vi "Abort.vi"   [LabVIEW 2023]
uses:
  <vilib>/eio/EIONode/EIONode.xnode
  <vilib>/rvi/DataTransferAndStorage/Container/XNode/niFpgaContainer.xnode
  <vilib>/rvi/DataTransferAndStorage/Register/Emulation/niFpgaRegisterEmulation.vi
  <vilib>/rvi/eio/common/nirviEmuTemplateMethod_errors.vi
types:
  T1 = cluster{bool, bool, bool, bool, bool, bool, bool, bool, bool, bool, bool, bool, bool, bool, bool, bool}
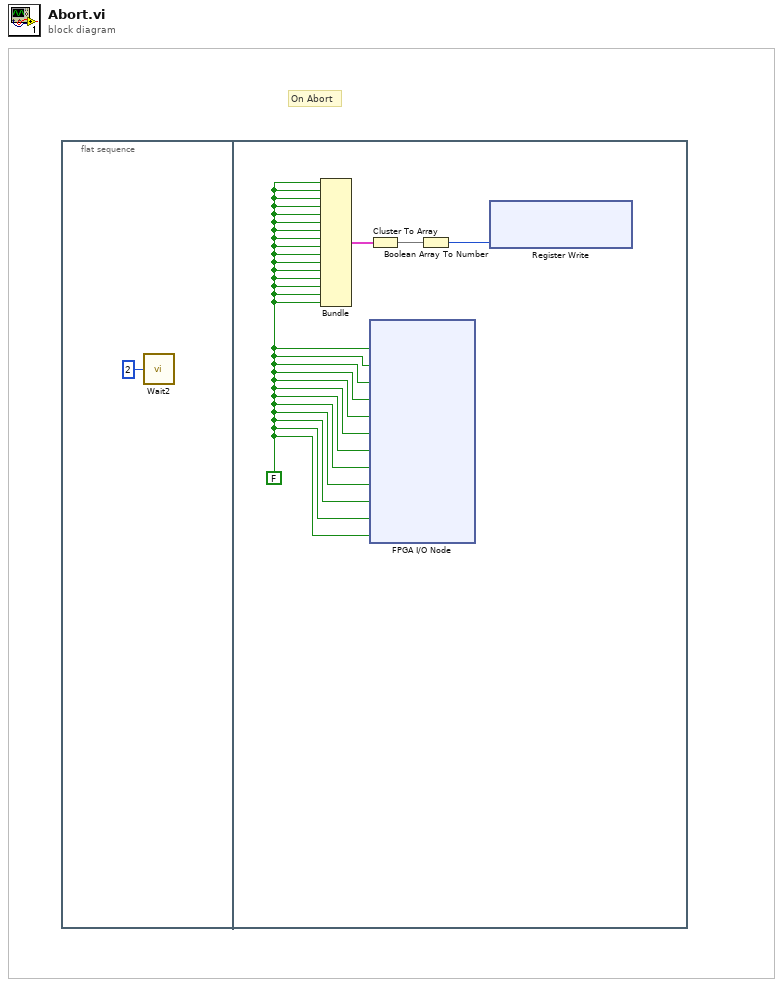
[diagram p0: block diagram]
diagram:
  # "On Abort"
  n1 = flat-sequence {
    frame #0 {
      n2 = call "Wait2"("Count(uSec)"=u8 2) -> ()  [unwired: 1 out]
    }
    frame #1 {
      w5 = FALSE
      n3 = Bundle(w5, w5, w5, w5, w5, w5, w5, w5, w5, w5, w5, w5, w5, w5, w5, w5) -> (w4:T1)  [unwired: 1 in]
      n4 = Cluster To Array(cluster=w4) -> (array=w3:bool[])
      n5 = xnode "FPGA I/O Node"("Mod2/DIO0"=w5, "Mod2/DIO1"=w5, "Mod2/DIO2"=w5, "Mod2/DIO3"=w5, "Mod3/DIO0"=w5, "Mod3/DIO1"=w5, "Mod3/DIO2"=w5, "Mod3/DIO3"=w5, "Mod4/DIO0"=w5, "Mod4/DIO1"=w5, "Mod4/DIO2"=w5, "Mod4/DIO3"=w5) -> ()  [unwired: 12 in, 12 out]
      n6 = Boolean Array To Number(Boolean array=w3) -> (number=w2:u16)
      n7 = xnode "Register Write"("Data"=w2) -> ()  [unwired: 1 in, 1 out]
    }
  }
